vi "Initialize.vi"(7 "Parcel Weight [kg]":dbl, 8 "error in (no error)":errorcluster, 9 "Recipient Data":T1, 10 "Sender Data":T1, 11 "Pigeon in":refnum<class "Pigeon.lvclass">) -> (0 "error out":errorcluster, 3 "Pigeon out":refnum<class "Pigeon.lvclass">)   [LabVIEW 2019, in "Pigeon.lvclass"]
uses:
  Pigeon.lvclass
  C:/Users/Extensa/Desktop/Fabryka/Fabryka Rozwiazanie/Delivery/Delivery/Delivery.lvclass
  Controls/#cluster_PersonalData.ctl
  Delivery/Delivery.lvclass/Delivery.ctl
  Delivery/Delivery.lvclass
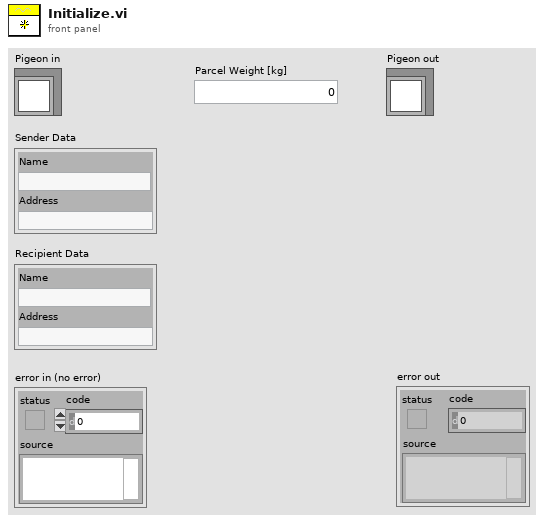
[diagram p1: front panel]
types:
  T1 = typedef "#cluster_PersonalData.ctl" = cluster{"Name":string, "Address":string}
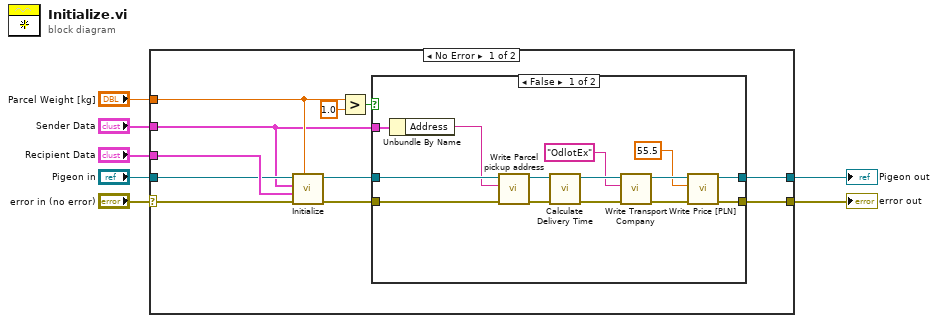
[diagram p0: block diagram]
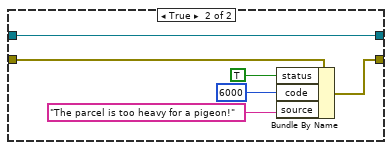
[diagram p2: hidden frame]
diagram:
  n1 = case shown="No Error" "error in (no error)" {
    selector: "error in (no error)" -> [w18 w39]
    tunnel: [w10 w39] -> w7
    tunnel: [w9 w40] -> w6
    tunnel: "Parcel Weight [kg]" -> [w15 _]
    tunnel: "Recipient Data" -> [w17 _]
    tunnel: "Sender Data" -> [w8 _]
    tunnel: "Pigeon in" -> [w16 w40]
    frame No Error {
      n2 = call-parent "Initialize.vi"("Parcel Weight [kg]"=w15, "error in (no error)"=w18, "Recipient Data"=w17, "Sender Data"=w8, "Delivery in"=w16) -> ("error out"=w13:errorcluster, "Delivery out"=w11:refnum<class "Pigeon.lvclass">)  [unwired: 5 in]
      n3 = Greater?(x=w15, y=1.0) -> (0:w12:bool)
      n4 = case shown="False" w12 {
        tunnel: w13 -> [w32 w38]
        tunnel: w11 -> [w31 w33]
        tunnel: [w20 w34] -> w10
        tunnel: [w21 w33] -> w9
        tunnel: w8 -> [w30 _]
        frame False {
          n5 = Unbundle By Name(w30) -> ("Address"=w29:string)
          n6 = call "Write Parcel pickup address.vi"("error in (no error)"=w32, "Parcel pickup address"=w29, "Delivery in"=w31) -> ("error out"=w28:errorcluster, "Delivery out"=w27:refnum<class "Pigeon.lvclass">)  [unwired: 7 in]
          n7 = call "Calculate Delivery Time.vi"("error in (no error)"=w28, "Pigeon in"=w27) -> ("error out"=w26:errorcluster, "Pigeon out"=w25:refnum<class "Pigeon.lvclass">)  [unwired: 8 in]
          n8 = call "Write Transport Company.vi"("error in (no error)"=w26, "Transport Company"="OdlotEx", "Delivery in"=w25) -> ("error out"=w23:errorcluster, "Delivery out"=w22:refnum<class "Pigeon.lvclass">)  [unwired: 7 in]
          n9 = call "Write Price [PLN].vi"("error in (no error)"=w23, "Price [PLN]"=55.5, "Delivery in"=w22) -> ("error out"=w20:errorcluster, "Delivery out"=w21:refnum<class "Pigeon.lvclass">)  [unwired: 7 in]
        }
        frame True {
          n10 = Bundle By Name(cluster=w38, "status"=TRUE, "code"=6000, "source"="The parcel is too heavy for a pigeon!") -> (w34:errorcluster)
        }
      }
    }
    frame Error {
    }
  }
  "error out" <- w7
  "Pigeon out" <- w6
